vi "ke37xx Configure Poles.vi"(0 "VISA Resource Name":refnum<visa-resource-name>, 1 "Channel List":string, 7 "Pole Setting":T1(ring), 11 "error in (no error)":errorcluster) -> (4 "VISA Resource Name Out":refnum<visa-resource-name>, 15 "error out":errorcluster)   [LabVIEW 2009, in "Keithley 3700 Series.lvlib"]
doc: "This VI allows you to configure the pole setting for the items specified in the Channel List control."
uses:
  <instrlib>/Keithley 3706/Keithley 3700 Series.lvlib
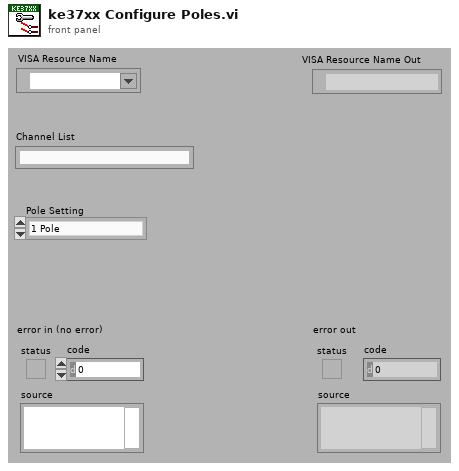
[diagram p1: front panel]
types:
  T1 = enum16{"1 Pole", "2 Pole", "3 Pole", "4 Pole", "6 Pole", ""}
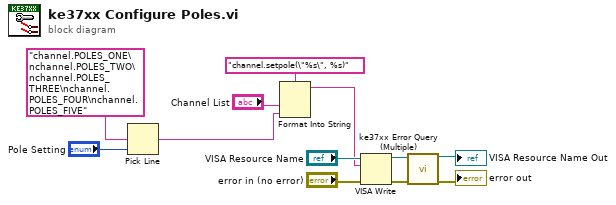
[diagram p0: block diagram]
diagram:
  n1 = Pick Line(multi-line string="channel.POLES_ONE\nchannel.POLES_TWO\nchannel.POLES_THREE\nchannel.POLES_FOUR\nchannel.POLES_FIVE", line index="Pole Setting") -> (output string=w2:string)  [unwired: 1 out]
  n2 = Format Into String(format string="channel.setpole(\"%s\", %s)", "Channel List", w2) -> (resulting string=w7:string)  [unwired: 2 in, 1 out]
  n3 = VISA Write(VISA resource name="VISA Resource Name", write buffer=w7, error in (no error)="error in (no error)") -> (VISA resource name out=w6:refnum<visa-resource-name>, error out=w5:errorcluster)  [unwired: 1 out]
  n4 = call <instrlib>:"ke37xx Error Query (Multiple).vi"("VISA resource name"=w6, "error in (no error)"=w5) -> ("VISA resource name out"=→"VISA Resource Name Out":refnum<visa-resource-name>, "error out"=→"error out":errorcluster)  [unwired: 12 out]
